vi "Dashboard Test.vi"() -> ()   [LabVIEW 2020, in "Visualisation.lvclass"]
uses:
  Visualisation.lvclass
  Application/Globals.vi
  Data Manager/Data Manager.lvclass
  Application/Application.lvlib
panel:
  out "Dist Name 24":string
  out "Dist Max 24":string
  out "Dist Name 23":string
  out "Dist Max 23":string
  out "Dist Max 22":string
  out "Dist Name 22":string
  out "Dist Name 21":string
  out "Dist Max 21":string
  out "Dist Max 20":string
  out "Dist Name 20":string
  out "Dist Max 19":string
  out "Dist Name 19":string
  out "A Walk 3":dbl format="%0.1f"
  out "B Walk 3":dbl format="%0.1f"
  out "B Run 3":dbl format="%0.1f"
  out "B Ride 3":dbl format="%0.1f"
  out "A Ride 9":dbl format="%0.1f"
  out "A Run 3":dbl format="%0.1f"
  out "Dist Max 18":dbl format="%<%H:%M:%S>t"
  out "Dist Name 18":string
  out "A Ride 8":dbl format="%<%H:%M:%S>t"
  out "Dist Max 17":dbl format="%<%H:%M:%S>t"
  out "Dist Name 17":string
  out "A Ride 7":dbl format="%<%H:%M:%S>t"
  out "Dist Max 16":dbl format="%<%H:%M:%S>t"
  out "Dist Name 16":string
  out "A Ride 6":dbl format="%<%H:%M:%S>t"
  out "Dist Max 15":dbl format="%<%H:%M:%S>t"
  out "Dist Name 15":string
  out "A Ride 5":dbl format="%<%H:%M:%S>t"
  out "Dist Max 14":dbl format="%<%H:%M:%S>t"
  out "Dist Name 14":string
  out "A Ride 4":dbl format="%<%H:%M:%S>t"
  out "Dist Max 13":dbl format="%<%H:%M:%S>t"
  out "Dist Name 13":string
  out "A Ride 3":dbl format="%<%H:%M:%S>t"
  out "A Walk 2":dbl
  out "B Walk 2":dbl
  out "B Run 2":dbl
  out "B Ride 2":dbl
  out "A Ride 2":dbl
  out "A Run 2":dbl
  out "Dist Name 12":string
  out "Dist Max 12":string
  out "Dist Name 11":string
  out "Dist Max 11":string
  out "Dist Max 10":string
  out "Dist Name 10":string
  out "Dist Name 9":string
  out "Dist Max 9":string
  out "Dist Max 8":string
  out "Dist Name 8":string
  out "Dist Max 7":string
  out "Dist Name 7":string
  out "Dist Name 6":string
  out "Dist Max 6":string
  out "Dist Name 5":string
  out "Dist Max 5":string
  out "Dist Max 4":string
  out "Dist Name 4":string
  out "Dist Name 3":string
  out "Dist Max 3":string
  out "Dist Name 2":string
  out "Dist Max 2":string
  out "Dist Max 1":string
  out "Dist Name 1":string
  out "B Ride":dbl format="%0.1f"
  out "B Run":dbl format="%0.1f"
  out "B Walk":dbl format="%0.1f"
  out "A Walk":dbl format="%0.1f"
  out "A Run":dbl format="%0.1f"
  out "A Ride":dbl format="%0.1f"
  out "B Total":dbl format="%0.1f km"
  out "A Total":dbl format="%0.1f km"
  out "Total Distance":dbl(slide) scale=-1.0..513.08705
  # "Total Activities"
  # "Total Distance (km)"
  # "Total Time"
  # "Total Elevation (m)"
  # "Team's Total"
  # "Team's Leader"
  # "Leader's Total"
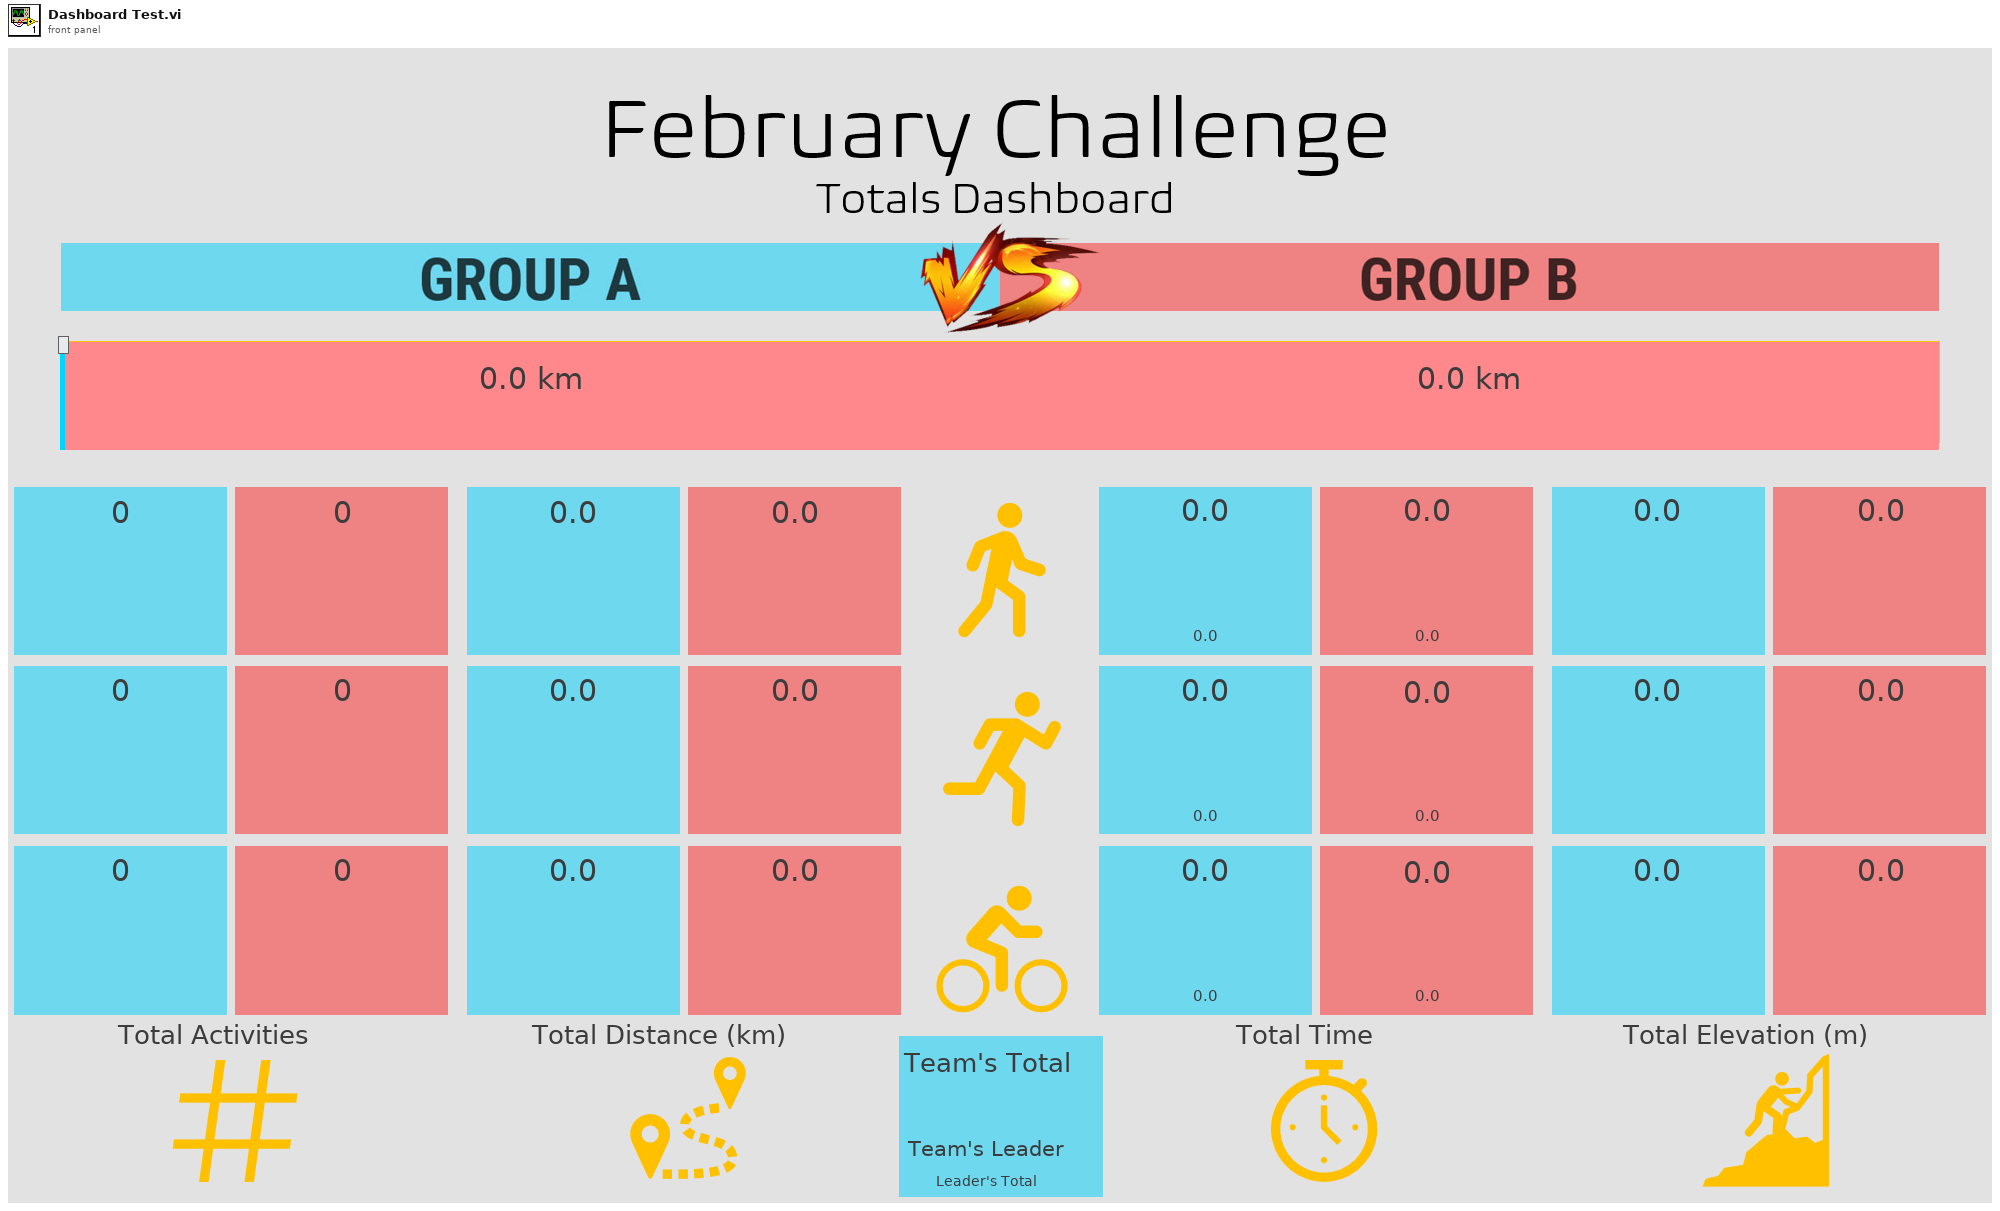
[diagram p1: front panel]
types:
  T1 = cluster{"Table":string[][], "Type":string, "Team":string}[]
  T2 = cluster{"Table":string[][], "Type":string, "Team":string}
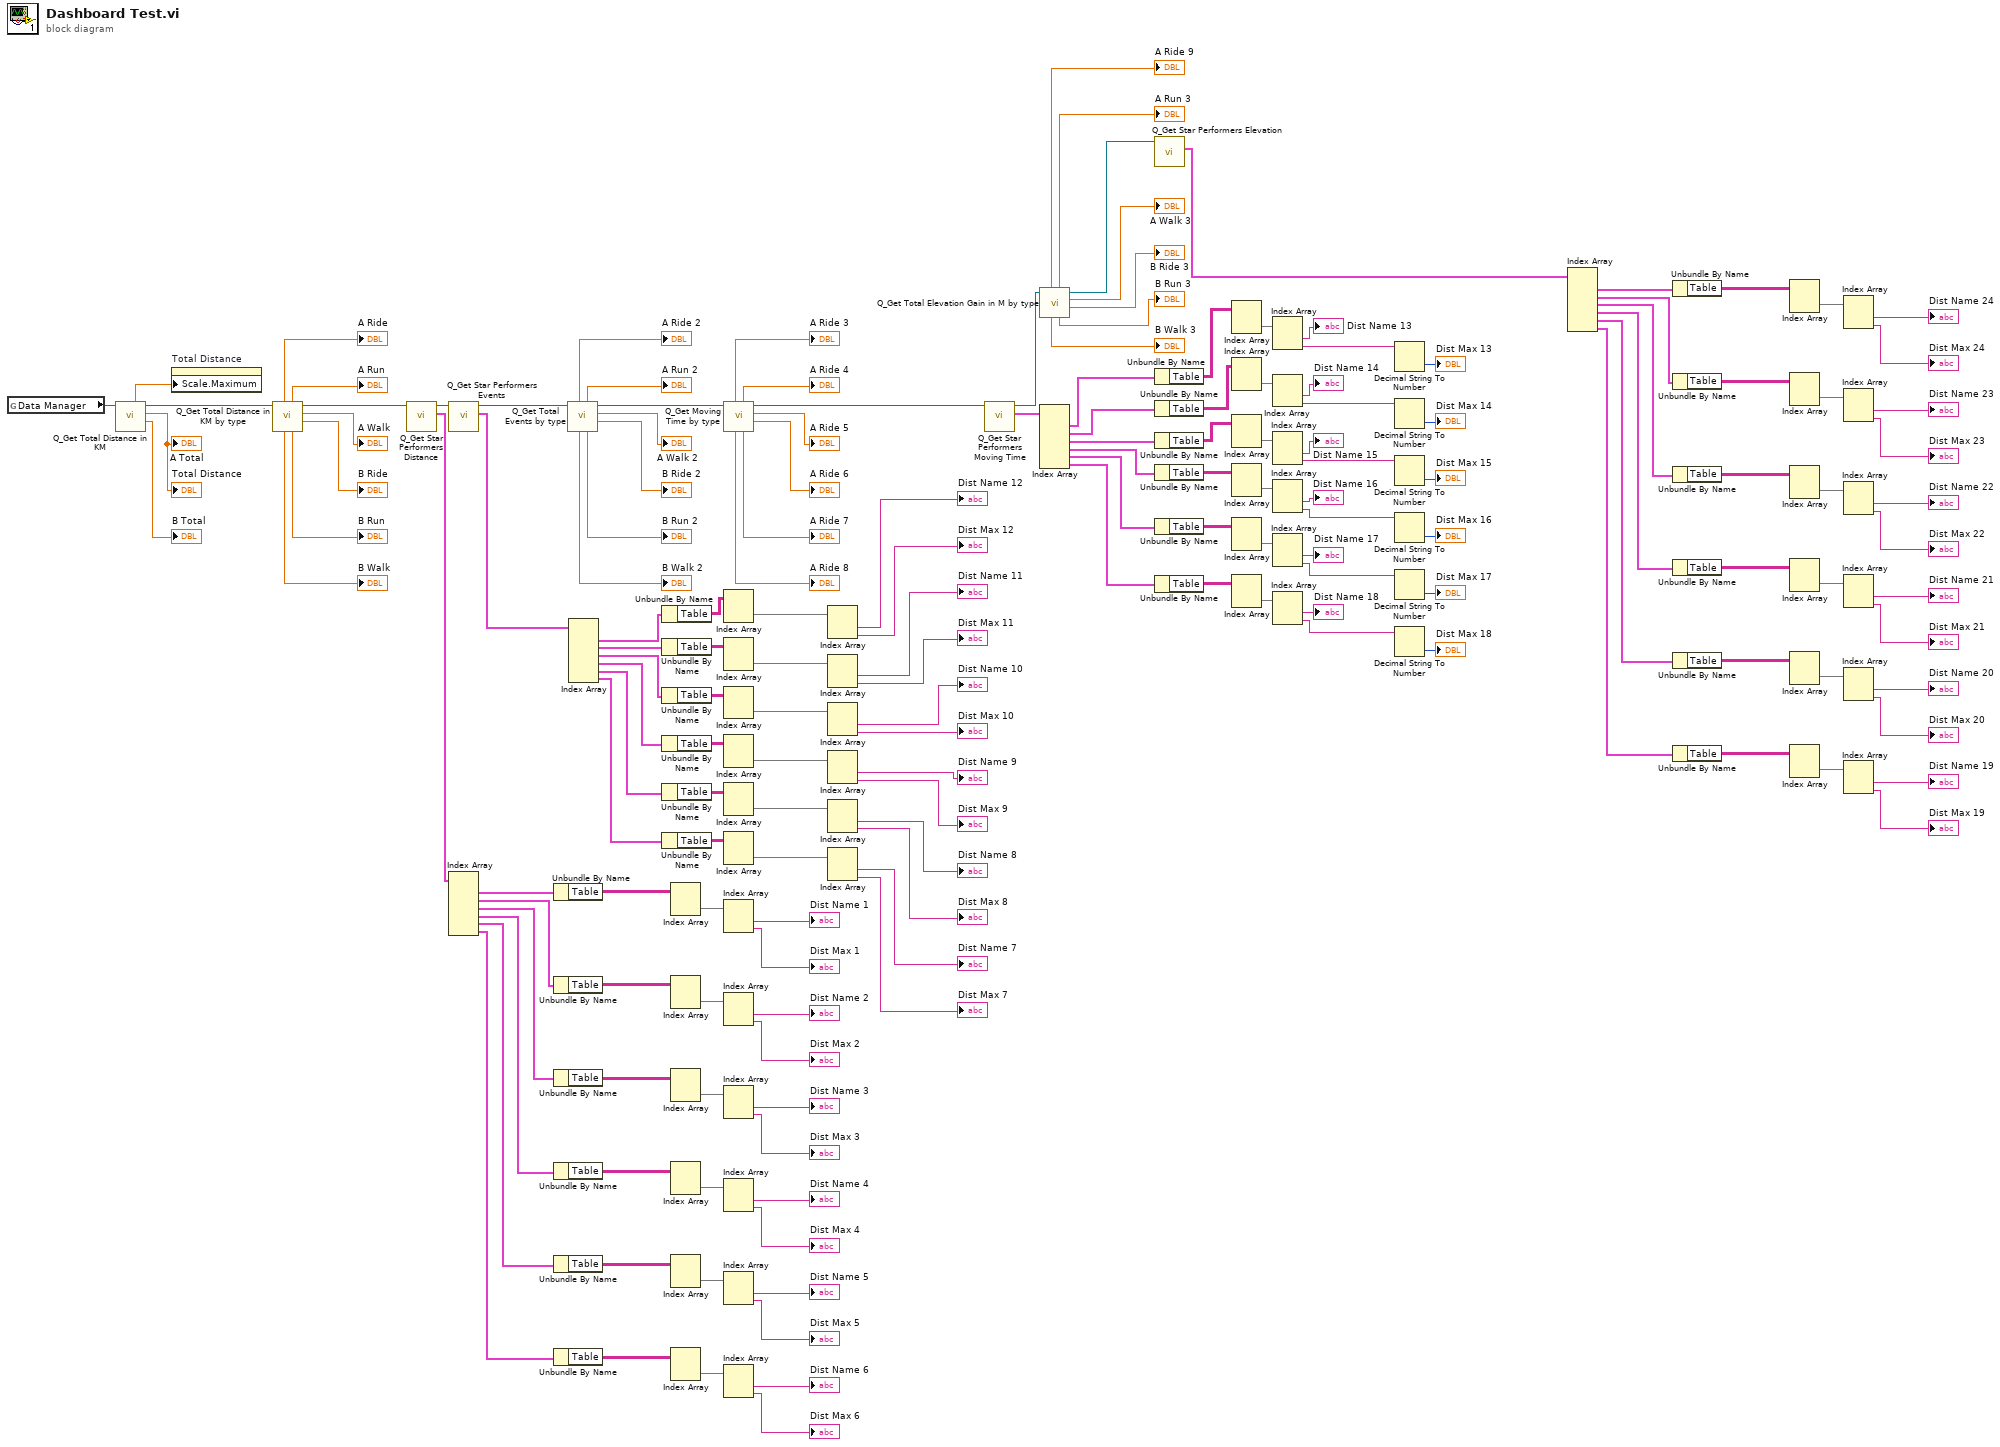
[diagram p0: block diagram]
diagram:
  n1 = global read "Globals.vi" "Data Manager"() -> (w166:refnum<class "Data Manager.lvclass">)
  n2 = call-dynamic "Q_Get Total Distance in KM.vi"("Data Manager in"=w166) -> ("Group B"=→"B Total":dbl, "Group A"=→"Total Distance" →"A Total":dbl, "Data Manager out"=w162:refnum<class "Data Manager.lvclass">, "Total"=w165:dbl)  [unwired: 6 in, 1 out]
  n3 = property on="Total Distance" class="Slide (strict)"("Scale.Maximum"=w165) -> ()  [unwired: 2 in, 2 out]
  n4 = call-dynamic "Q_Get Total Distance in KM by type.vi"("Data Manager in"=w162) -> ("B Ride"=→"B Ride":dbl, "A Walk"=→"A Walk":dbl, "Data Manager out"=w155:refnum<class "Data Manager.lvclass">, "Run"=→"B Run":dbl, "A Run"=→"A Run":dbl, "Walk"=→"B Walk":dbl, "A Ride"=→"A Ride":dbl)  [unwired: 3 in, 1 out]
  n5 = call-dynamic "Q_Get Star Performers Distance.vi"("Data Manager in"=w155) -> ("All Tables"=w124:T1, "Data Manager out"=w123:refnum<class "Data Manager.lvclass">)  [unwired: 8 in, 1 out]
  n6 = call-dynamic "Q_Get Star Performers Events.vi"("Data Manager in"=w123) -> ("All Tables"=w92:T1, "Data Manager out"=w91:refnum<class "Data Manager.lvclass">)  [unwired: 8 in, 1 out]
  n7 = Index Array(array=w124) -> (element #1=w154:T2, element #2=w145:T2, element #3=w142:T2, element #4=w133:T2, element #5=w132:T2, element #6=w131:T2)  [unwired: 6 in]
  n8 = Unbundle By Name(w154) -> ("Table"=w153:string[][])
  n9 = Unbundle By Name(w145) -> ("Table"=w146:string[][])
  n10 = Unbundle By Name(w142) -> ("Table"=w144:string[][])
  n11 = Unbundle By Name(w133) -> ("Table"=w134:string[][])
  n12 = Unbundle By Name(w132) -> ("Table"=w137:string[][])
  n13 = Unbundle By Name(w131) -> ("Table"=w138:string[][])
  n14 = call-dynamic "Q_Get Total Events by type.vi"("Data Manager in"=w91) -> ("B Ride"=→"B Ride 2":dbl, "A Walk"=→"A Walk 2":dbl, "Data Manager out"=w84:refnum<class "Data Manager.lvclass">, "Run"=→"B Run 2":dbl, "A Run"=→"A Run 2":dbl, "Walk"=→"B Walk 2":dbl, "A Ride"=→"A Ride 2":dbl)  [unwired: 3 in, 1 out]
  n15 = Index Array(array=w92) -> (element #1=w93:T2, element #2=w102:T2, element #3=w105:T2, element #4=w114:T2, element #5=w115:T2, element #6=w116:T2)  [unwired: 6 in]
  n16 = Unbundle By Name(w93) -> ("Table"=w94:string[][])
  n17 = Unbundle By Name(w102) -> ("Table"=w101:string[][])
  n18 = Unbundle By Name(w105) -> ("Table"=w103:string[][])
  n19 = Unbundle By Name(w114) -> ("Table"=w113:string[][])
  n20 = Unbundle By Name(w115) -> ("Table"=w110:string[][])
  n21 = Unbundle By Name(w116) -> ("Table"=w109:string[][])
  n22 = Index Array(array=w153) -> (element=w152:string[])  [unwired: 2 in]
  n23 = Index Array(array=w146) -> (element=w147:string[])  [unwired: 2 in]
  n24 = Index Array(array=w144) -> (element=w143:string[])  [unwired: 2 in]
  n25 = Index Array(array=w134) -> (element=w135:string[])  [unwired: 2 in]
  n26 = Index Array(array=w137) -> (element=w136:string[])  [unwired: 2 in]
  n27 = Index Array(array=w138) -> (element=w139:string[])  [unwired: 2 in]
  n28 = call-dynamic "Q_Get Moving Time by type.vi"("Data Manager in"=w84) -> ("B Ride"=→"A Ride 6":dbl, "A Walk"=→"A Ride 5":dbl, "Data Manager out"=w83:refnum<class "Data Manager.lvclass">, "Run"=→"A Ride 7":dbl, "A Run"=→"A Ride 4":dbl, "Walk"=→"A Ride 8":dbl, "A Ride"=→"A Ride 3":dbl)  [unwired: 3 in, 1 out]
  n29 = Index Array(array=w94) -> (element=w95:string[])  [unwired: 2 in]
  n30 = Index Array(array=w101) -> (element=w100:string[])  [unwired: 2 in]
  n31 = Index Array(array=w103) -> (element=w104:string[])  [unwired: 2 in]
  n32 = Index Array(array=w113) -> (element=w112:string[])  [unwired: 2 in]
  n33 = Index Array(array=w110) -> (element=w111:string[])  [unwired: 2 in]
  n34 = Index Array(array=w109) -> (element=w108:string[])  [unwired: 2 in]
  n35 = Index Array(array=w152) -> (element #1=→"Dist Name 1":string, element #2=→"Dist Max 1":string)  [unwired: 2 in]
  n36 = Index Array(array=w147) -> (element #1=→"Dist Name 2":string, element #2=→"Dist Max 2":string)  [unwired: 2 in]
  n37 = Index Array(array=w143) -> (element #1=→"Dist Name 3":string, element #2=→"Dist Max 3":string)  [unwired: 2 in]
  n38 = Index Array(array=w135) -> (element #1=→"Dist Name 4":string, element #2=→"Dist Max 4":string)  [unwired: 2 in]
  n39 = Index Array(array=w136) -> (element #1=→"Dist Name 5":string, element #2=→"Dist Max 5":string)  [unwired: 2 in]
  n40 = Index Array(array=w139) -> (element #1=→"Dist Name 6":string, element #2=→"Dist Max 6":string)  [unwired: 2 in]
  n41 = Index Array(array=w95) -> (element #1=→"Dist Name 12":string, element #2=→"Dist Max 12":string)  [unwired: 2 in]
  n42 = Index Array(array=w100) -> (element #1=→"Dist Name 11":string, element #2=→"Dist Max 11":string)  [unwired: 2 in]
  n43 = Index Array(array=w104) -> (element #1=→"Dist Name 10":string, element #2=→"Dist Max 10":string)  [unwired: 2 in]
  n44 = Index Array(array=w112) -> (element #1=→"Dist Name 9":string, element #2=→"Dist Max 9":string)  [unwired: 2 in]
  n45 = Index Array(array=w111) -> (element #1=→"Dist Name 8":string, element #2=→"Dist Max 8":string)  [unwired: 2 in]
  n46 = Index Array(array=w108) -> (element #1=→"Dist Name 7":string, element #2=→"Dist Max 7":string)  [unwired: 2 in]
  n47 = call-dynamic "Q_Get Star Performers Moving Time.vi"("Data Manager in"=w83) -> ("All Tables"=w79:T1, "Data Manager out"=w39:refnum<class "Data Manager.lvclass">)  [unwired: 8 in, 1 out]
  n48 = call-dynamic "Q_Get Total Elevation Gain in M by type.vi"("Data Manager in"=w39) -> ("B Ride"=→"B Ride 3":dbl, "A Walk"=→"A Walk 3":dbl, "Data Manager out"=w38:refnum<class "Data Manager.lvclass">, "Run"=→"B Run 3":dbl, "A Run"=→"A Run 3":dbl, "Walk"=→"B Walk 3":dbl, "A Ride"=→"A Ride 9":dbl)  [unwired: 3 in, 1 out]
  n49 = Index Array(array=w79) -> (element #1=w82:T2, element #2=w54:T2, element #3=w53:T2, element #4=w52:T2, element #5=w51:T2, element #6=w50:T2)  [unwired: 6 in]
  n50 = call-dynamic "Q_Get Star Performers Elevation.vi"("Data Manager in"=w38) -> ("All Tables"=w1:T1)  [unwired: 8 in, 2 out]
  n51 = Unbundle By Name(w82) -> ("Table"=w81:string[][])
  n52 = Unbundle By Name(w54) -> ("Table"=w67:string[][])
  n53 = Unbundle By Name(w53) -> ("Table"=w66:string[][])
  n54 = Unbundle By Name(w52) -> ("Table"=w61:string[][])
  n55 = Unbundle By Name(w51) -> ("Table"=w60:string[][])
  n56 = Unbundle By Name(w50) -> ("Table"=w55:string[][])
  n57 = Index Array(array=w81) -> (element=w80:string[])  [unwired: 2 in]
  n58 = Index Array(array=w67) -> (element=w68:string[])  [unwired: 2 in]
  n59 = Index Array(array=w66) -> (element=w65:string[])  [unwired: 2 in]
  n60 = Index Array(array=w61) -> (element=w62:string[])  [unwired: 2 in]
  n61 = Index Array(array=w60) -> (element=w59:string[])  [unwired: 2 in]
  n62 = Index Array(array=w55) -> (element=w56:string[])  [unwired: 2 in]
  n63 = Index Array(array=w80) -> (element #1=→"Dist Name 13":string, element #2=w77:string)  [unwired: 2 in]
  n64 = Index Array(array=w68) -> (element #1=→"Dist Name 14":string, element #2=w69:string)  [unwired: 2 in]
  n65 = Index Array(array=w65) -> (element #1=→"Dist Name 15":string, element #2=w64:string)  [unwired: 2 in]
  n66 = Index Array(array=w62) -> (element #1=→"Dist Name 16":string, element #2=w63:string)  [unwired: 2 in]
  n67 = Index Array(array=w59) -> (element #1=→"Dist Name 17":string, element #2=w58:string)  [unwired: 2 in]
  n68 = Index Array(array=w56) -> (element #1=→"Dist Name 18":string, element #2=w57:string)  [unwired: 2 in]
  n69 = Decimal String To Number(string=w77) -> (number=→"Dist Max 13":i32)  [unwired: 2 in, 1 out]
  n70 = Decimal String To Number(string=w69) -> (number=→"Dist Max 14":i32)  [unwired: 2 in, 1 out]
  n71 = Decimal String To Number(string=w64) -> (number=→"Dist Max 15":i32)  [unwired: 2 in, 1 out]
  n72 = Decimal String To Number(string=w63) -> (number=→"Dist Max 16":i32)  [unwired: 2 in, 1 out]
  n73 = Decimal String To Number(string=w58) -> (number=→"Dist Max 17":i32)  [unwired: 2 in, 1 out]
  n74 = Decimal String To Number(string=w57) -> (number=→"Dist Max 18":i32)  [unwired: 2 in, 1 out]
  n75 = Index Array(array=w1) -> (element #1=w2:T2, element #2=w11:T2, element #3=w14:T2, element #4=w23:T2, element #5=w24:T2, element #6=w25:T2)  [unwired: 6 in]
  n76 = Unbundle By Name(w2) -> ("Table"=w3:string[][])
  n77 = Unbundle By Name(w11) -> ("Table"=w10:string[][])
  n78 = Unbundle By Name(w14) -> ("Table"=w12:string[][])
  n79 = Unbundle By Name(w23) -> ("Table"=w22:string[][])
  n80 = Unbundle By Name(w24) -> ("Table"=w19:string[][])
  n81 = Unbundle By Name(w25) -> ("Table"=w18:string[][])
  n82 = Index Array(array=w3) -> (element=w4:string[])  [unwired: 2 in]
  n83 = Index Array(array=w10) -> (element=w9:string[])  [unwired: 2 in]
  n84 = Index Array(array=w12) -> (element=w13:string[])  [unwired: 2 in]
  n85 = Index Array(array=w22) -> (element=w21:string[])  [unwired: 2 in]
  n86 = Index Array(array=w19) -> (element=w20:string[])  [unwired: 2 in]
  n87 = Index Array(array=w18) -> (element=w17:string[])  [unwired: 2 in]
  n88 = Index Array(array=w4) -> (element #1=→"Dist Name 24":string, element #2=→"Dist Max 24":string)  [unwired: 2 in]
  n89 = Index Array(array=w9) -> (element #1=→"Dist Name 23":string, element #2=→"Dist Max 23":string)  [unwired: 2 in]
  n90 = Index Array(array=w13) -> (element #1=→"Dist Name 22":string, element #2=→"Dist Max 22":string)  [unwired: 2 in]
  n91 = Index Array(array=w21) -> (element #1=→"Dist Name 21":string, element #2=→"Dist Max 21":string)  [unwired: 2 in]
  n92 = Index Array(array=w20) -> (element #1=→"Dist Name 20":string, element #2=→"Dist Max 20":string)  [unwired: 2 in]
  n93 = Index Array(array=w17) -> (element #1=→"Dist Name 19":string, element #2=→"Dist Max 19":string)  [unwired: 2 in]
